vi "Sos_Kv_2024.vi"(0 "Type of air":i32(listbox)=4, 1 "Temperature (K)":dbl=293.4405 format="%.4g", 2 "Pressure (Pa)":dbl=99951.0 format="%.3f", 3 "CO2 content (ppm)":dbl=542.0, 4 "xw molar fraction water vapor":dbl=0.013091 format="%.6g") -> (5 "Sos Kv (m/s)":dbl=344.20109788026724 format="%.4g", 6 "Kv":dbl=0.0005394017882816821)   [LabVIEW 2016]
panel:
  out "Kv (ppm)":dbl=539.4017882816821 format="%.1f"
  out "Sos gamma0RT/M check [m/s]":dbl=344.1083040745762 format="%.4g"
  out "sos Kc [m/s]":dbl=344.1083040745762 format="%.4f"
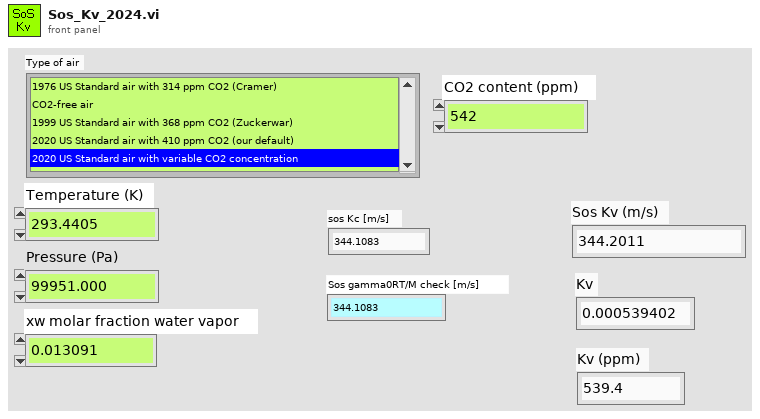
[diagram p1: front panel]
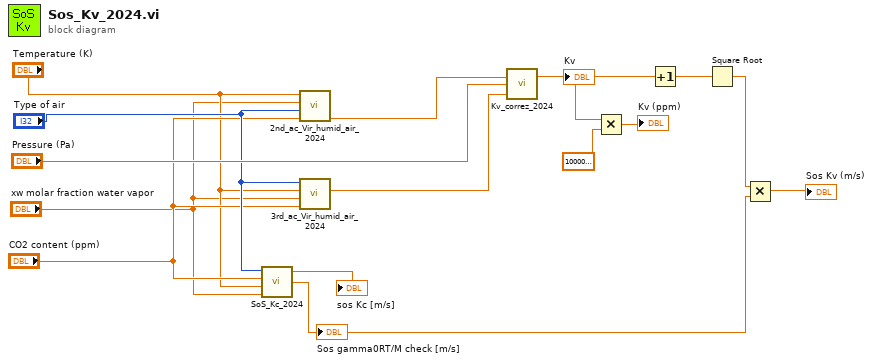
[diagram p0: block diagram]
diagram:
  n1 = call "SoS_Kc_2024.vi"("xw H2O molar fraction"="xw molar fraction water vapor", "Temperature [K]"="Temperature (K)", "CO2 content (ppm)"="CO2 content (ppm)", "Type of air"="Type of air") -> ("Sos gamma0RT/M check [m/s]"=w4:dbl, "Sos Kc (m/s)"=→"sos Kc [m/s]":dbl)  [unwired: 1 out]
  "Sos gamma0RT/M check [m/s]" <- w4
  n2 = call "2nd_ac_Vir_humid_air_2024.vi"("CO2 content (ppm)"="CO2 content (ppm)", "Type of air"="Type of air", "xw molar fraction water vapor"="xw molar fraction water vapor", "Temperature (K)"="Temperature (K)") -> ("2nd ac pressure vir humid air b or \"F\""=w13:dbl)  [unwired: 3 out]
  n3 = call "3rd_ac_Vir_humid_air_2024.vi"("CO2 content (ppm)"="CO2 content (ppm)", "Water Vapor Mole Fraction"="xw molar fraction water vapor", "Temperature [K]"="Temperature (K)", "Type of air"="Type of air") -> ("3rd ac press Virial [G]"=w12:dbl)  [unwired: 2 in, 5 out]
  n4 = call "Kv_correz_2024.vi"("3rd ac pressure Virial \"G\" (Pa^-2)"=w12, "Pressure [Pa]"="Pressure (Pa)", "2nd ac pressure Virial \"F\" (Pa^-1)"=w13) -> ("Kv"=w3:dbl)  [unwired: 1 in]
  "Kv" <- w3
  n5 = Multiply(x=w3, y=1000000.0) -> (x*y=→"Kv (ppm)":dbl)
  n6 = Increment(x=w3) -> (x+1=w14:dbl)
  n7 = Square Root(x=w14) -> (sqrt(x)=w5:dbl)
  n8 = Multiply(x=w5, y=w4) -> (x*y=→"Sos Kv (m/s)":dbl)
